vi "Check if frame available.vi"(8 "error in (no error)":errorcluster, 11 "camera handle in":i16) -> (0 "error out":errorcluster, 2 "is frame ready?":bool, 3 "camera handle out":i16)   [LabVIEW 2012]
uses:
  Visual Studio/Cascade wrapper/Release/Cascade wrapper.dll
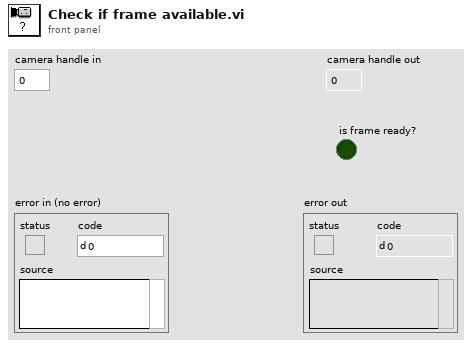
[diagram p1: front panel]
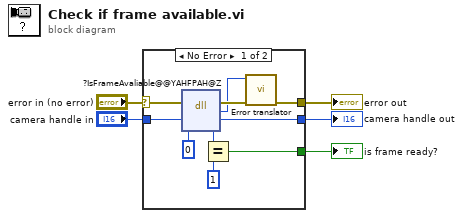
[diagram p0: block diagram]
diagram:
  n1 = case shown="No Error" "error in (no error)" {
    selector: "error in (no error)" -> [w15 w17]
    tunnel: "camera handle in" -> [w14 w16]
    tunnel: [w11 w16] -> w3
    tunnel: [w10 w17] -> w2
    tunnel: [w6 _] -> w1
    frame No Error {
      n2 = dll-call lib="C:/moroder/Cascade wrapper/Visual Studio/Cascade wrapper/Release/Cascade wrapper.dll" fn="?IsFrameAvaliable@@YAHFPAH@Z"(error in=w15, "camera handle"=w14, "status"=0) -> (error out=w13:errorcluster, "error"=w12:i32, "camera handle"=w11:i16, "status"=w8:i32)  [unwired: 2 in, 1 out]
      n3 = Equal?(x=w8, y=1) -> (x = y?=w6:bool)
      n4 = call "Error translator.vi"("error in (no error)"=w13, "error code"=w12) -> ("error out"=w10:errorcluster)  [unwired: 9 in]
    }
    frame Error {
    }
  }
  "error out" <- w2
  "camera handle out" <- w3
  "is frame ready?" <- w1
